vi "PropertyNodes.vi"() -> ()   [LabVIEW 2018]
panel:
  out "?":string
  in  "?":bool
  # "Blue"
  # "Green"
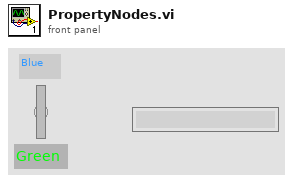
[diagram p1: front panel]
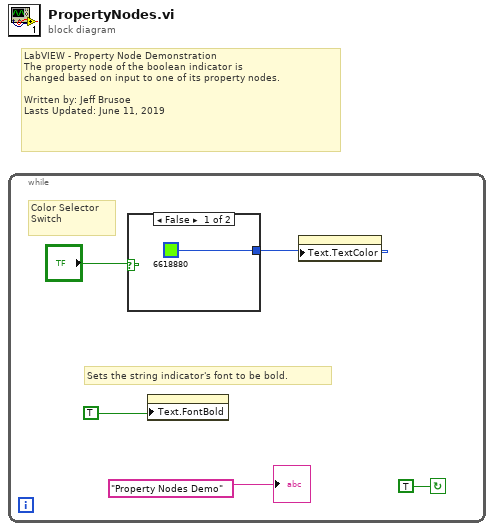
[diagram p0: block diagram]
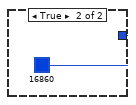
[diagram p2: hidden frame]
diagram:
  # "LabVIEW - Property Node Demonstration\nThe property node of the boolean indicator is\nchanged based on input to one of its property nodes.\n\nWritten by: Jeff Brusoe\nLasts Updated: June 11, 2019"
  n1 = while {
    stop <- TRUE continue-if-true
    # "Color Selector\nSwitch"
    # "Sets the string indicator's font to be bold."
    n2 = case shown="False" "?" {
      tunnel: [u32 6618880 u32 16860] -> w3
      frame False {
      }
      frame True {
      }
    }
    n3 = property class="Str"("Text.FontBold"=TRUE) -> ()  [unwired: 2 in, 2 out]
    n4 = property class="Str"("Text.TextColor"=w3) -> ()  [unwired: 2 in, 2 out]
    "?" <- "Property Nodes Demo"
  }
